vi "OnAxisPotential.vi"(1 "Requested Excitations":dbl[](array[numeric])=[0.0, 10.0, 10.0, 2.0, 20.0, 0.0, 0.0, 0.0, 0.0, 0.0, 0.0, 0.0, 0.0, 0.0, 0.0, 0.0, 0.0, 0.0, 0.0, 0.0, 0.0, 0.0], 2 "ComsolArray":dbl[][](array[numeric])=array1050x22[23100 elements], 3 "z (m)":dbl[](array[numeric])=[-0.5004, -0.4999, -0.4995, -0.499, -0.4985, -0.498, -0.4975, -0.4971, -0.4966, -0.4961, -0.4956, -0.4952, -0.4947, -0.4942, -0.4937, -0.4933, -0.4928, -0.4923, -0.4918, -0.4913, -0.4909, -0.4904, -0.4899, -0.4894, -0.489, -0.4885, -0.488, -0.4875, -0.4871, -0.4866, -0.4861, -0.4856, -0.4851, -0.4847, -0.4842, -0.4837, -0.4832, -0.4828, -0.4823, -0.4818, -0.4813, -0.4809, -0.4804, -0.4799, -0.4794, -0.4789, -0.4785, -0.478, -0.4775, -0.477, -0.4766, -0.4761, -0.4756, -0.4751, -0.4747, -0.4742, -0.4737, -0.4732, -0.4727, -0.4723, -0.4718, -0.4713, -0.4708, -0.4704, -0.4699, -0.4694, -0.4689, -0.4685, -0.468, -0.4675, -0.467, -0.4665, -0.4661, -0.4656, -0.4651, -0.4646, -0.4642, -0.4637, -0.4632, -0.4627, -0.4623, -0.4618, -0.4613, -0.4608, -0.4604, -0.4599, -0.4594, -0.4589, -0.4584, -0.458, -0.4575, -0.457, -0.4565, -0.4561, -0.4556, -0.4551, -0.4546, -0.4542, -0.4537, -0.4532, -0.4527, -0.4522, -0.4518, -0.4513, -0.4508, -0.4503, -0.4499, -0.4494, -0.4489, -0.4484, -0.448, -0.4475, -0.447, -0.4465, -0.446, -0.4456, -0.4451, -0.4446, -0.4441, -0.4437, -0.4432, -0.4427, -0.4422, -0.4418, -0.4413, -0.4408, -0.4403, -0.4398, -0.4394, -0.4389, -0.4384, -0.4379, -0.4375, -0.437, -0.4365, -0.436, -0.4356, -0.4351, -0.4346, -0.4341, -0.4336, -0.4332, -0.4327, -0.4322, -0.4317, -0.4313, -0.4308, -0.4303, -0.4298, -0.4294, -0.4289, -0.4284, -0.4279, -0.4274, -0.427, -0.4265, -0.426, -0.4255, -0.4251, -0.4246, -0.4241, -0.4236, -0.4232, -0.4227, -0.4222, -0.4217, -0.4212, -0.4208, -0.4203, -0.4198, -0.4193, -0.4189, -0.4184, -0.4179, -0.4174, -0.417, -0.4165, -0.416, -0.4155, -0.415, -0.4146, -0.4141, -0.4136, -0.4131, -0.4127, -0.4122, -0.4117, -0.4112, -0.4108, -0.4103, -0.4098, -0.4093, -0.4089, -0.4084, -0.4079, -0.4074, -0.4069, -0.4065, -0.406, -0.4055, -0.405, -0.4046, -0.4041, -0.4036, -0.4031, -0.4027, -0.4022, -0.4017, -0.4012, -0.4007, -0.4003, -0.3998, -0.3993, -0.3988, -0.3984, -0.3979, -0.3974, -0.3969, -0.3965, -0.396, -0.3955, -0.395, -0.3945, -0.3941, -0.3936, -0.3931, -0.3926, -0.3922, -0.3917, -0.3912, -0.3907, -0.3903, -0.3898, -0.3893, -0.3888, -0.3883, -0.3879, -0.3874, -0.3869, -0.3864, -0.386, -0.3855, -0.385, -0.3845, -0.3841, -0.3836, -0.3831, -0.3826, -0.3821, -0.3817, -0.3812, -0.3807, -0.3802, -0.3798, -0.3793, -0.3788, -0.3783, -0.3779, -0.3774, -0.3769, -0.3764, -0.3759, -0.3755, -0.375, -0.3745, -0.374, -0.3736, -0.3731, -0.3726, -0.3721, -0.3717, -0.3712, -0.3707, -0.3702, -0.3697, -0.3693, -0.3688, -0.3683, -0.3678, -0.3674, -0.3669, -0.3664, -0.3659, -0.3655, -0.365, -0.3645, -0.364, -0.3635, -0.3631, -0.3626, -0.3621, -0.3616, -0.3612, -0.3607, -0.3602, -0.3597, -0.3593, -0.3588, -0.3583, -0.3578, -0.3573, -0.3569, -0.3564, -0.3559, -0.3554, -0.355, -0.3545, -0.354, -0.3535, -0.3531, -0.3526, -0.3521, -0.3516, -0.3512, -0.3507, -0.3502, -0.3497, -0.3492, -0.3488, -0.3483, -0.3478, -0.3473, -0.3469, -0.3464, -0.3459, -0.3454, -0.345, -0.3445, -0.344, -0.3435, -0.343, -0.3426, -0.3421, -0.3416, -0.3411, -0.3407, -0.3402, -0.3397, -0.3392, -0.3388, -0.3383, -0.3378, -0.3373, -0.3368, -0.3364, -0.3359, -0.3354, -0.3349, -0.3345, -0.334, -0.3335, -0.333, -0.3326, -0.3321, -0.3316, -0.3311, -0.3306, -0.3302, -0.3297, -0.3292, -0.3287, -0.3283, -0.3278, -0.3273, -0.3268, -0.3264, -0.3259, -0.3254, -0.3249, -0.3244, -0.324, -0.3235, -0.323, -0.3225, -0.3221, -0.3216, -0.3211, -0.3206, -0.3202, -0.3197, -0.3192, -0.3187, -0.3182, -0.3178, -0.3173, -0.3168, -0.3163, -0.3159, -0.3154, -0.3149, -0.3144, -0.314, -0.3135, -0.313, -0.3125, -0.3121, -0.3116, -0.3111, -0.3106, -0.3101, -0.3097, -0.3092, -0.3087, -0.3082, -0.3078, -0.3073, -0.3068, -0.3063, -0.3059, -0.3054, -0.3049, -0.3044, -0.3039, -0.3035, -0.303, -0.3025, -0.302, -0.3016, -0.3011, -0.3006, -0.3001, -0.2997, -0.2992, -0.2987, -0.2982, -0.2977, -0.2973, -0.2968, -0.2963, -0.2958, -0.2954, -0.2949, -0.2944, -0.2939, -0.2935, -0.293, -0.2925, -0.292, -0.2915, -0.2911, -0.2906, -0.2901, -0.2896, -0.2892, -0.2887, -0.2882, -0.2877, -0.2873, -0.2868, -0.2863, -0.2858, -0.2853, -0.2849, -0.2844, -0.2839, -0.2834, -0.283, -0.2825, -0.282, -0.2815, -0.2811, -0.2806, -0.2801, -0.2796, -0.2791, -0.2787, -0.2782, -0.2777, -0.2772, -0.2768, -0.2763, -0.2758, -0.2753, -0.2749, -0.2744, -0.2739, -0.2734, -0.2729, -0.2725, -0.272, -0.2715, -0.271, -0.2706, -0.2701, -0.2696, -0.2691, -0.2687, -0.2682, -0.2677, -0.2672, -0.2667, -0.2663, -0.2658, -0.2653, -0.2648, -0.2644, -0.2639, -0.2634, -0.2629, -0.2625, -0.262, -0.2615, -0.261, -0.2605, -0.2601, -0.2596, -0.2591, -0.2586, -0.2582, -0.2577, -0.2572, -0.2567, -0.2563, -0.2558, -0.2553, -0.2548, -0.2544, -0.2539, -0.2534, -0.2529, -0.2524, -0.252, -0.2515, -0.251, -0.2505, -0.2501, -0.2496, -0.2491, -0.2486, -0.2482, -0.2477, -0.2472, -0.2467, -0.2462, -0.2458, -0.2453, -0.2448, -0.2443, -0.2439, -0.2434, -0.2429, -0.2424, -0.242, -0.2415, -0.241, -0.2405, -0.24, -0.2396, -0.2391, -0.2386, -0.2381, -0.2377, -0.2372, -0.2367, -0.2362, -0.2358, -0.2353, -0.2348, -0.2343, -0.2338, -0.2334, -0.2329, -0.2324, -0.2319, -0.2315, -0.231, -0.2305, -0.23, -0.2296, -0.2291, -0.2286, -0.2281, -0.2276, -0.2272, -0.2267, -0.2262, -0.2257, -0.2253, -0.2248, -0.2243, -0.2238, -0.2234, -0.2229, -0.2224, -0.2219, -0.2214, -0.221, -0.2205, -0.22, -0.2195, -0.2191, -0.2186, -0.2181, -0.2176, -0.2172, -0.2167, -0.2162, -0.2157, -0.2153, -0.2148, -0.2143, -0.2138, -0.2133, -0.2129, -0.2124, -0.2119, -0.2114, -0.211, -0.2105, -0.21, -0.2095, -0.2091, -0.2086, -0.2081, -0.2076, -0.2071, -0.2067, -0.2062, -0.2057, -0.2052, -0.2048, -0.2043, -0.2038, -0.2033, -0.2029, -0.2024, -0.2019, -0.2014, -0.2009, -0.2005, -0.2, -0.1995, -0.199, -0.1986, -0.1981, -0.1976, -0.1971, -0.1967, -0.1962, -0.1957, -0.1952, -0.1947, -0.1943, -0.1938, -0.1933, -0.1928, -0.1924, -0.1919, -0.1914, -0.1909, -0.1905, -0.19, -0.1895, -0.189, -0.1885, -0.1881, -0.1876, -0.1871, -0.1866, -0.1862, -0.1857, -0.1852, -0.1847, -0.1843, -0.1838, -0.1833, -0.1828, -0.1823, -0.1819, -0.1814, -0.1809, -0.1804, -0.18, -0.1795, -0.179, -0.1785, -0.1781, -0.1776, -0.1771, -0.1766, -0.1761, -0.1757, -0.1752, -0.1747, -0.1742, -0.1738, -0.1733, -0.1728, -0.1723, -0.1719, -0.1714, -0.1709, -0.1704, -0.1699, -0.1695, -0.169, -0.1685, -0.168, -0.1676, -0.1671, -0.1666, -0.1661, -0.1657, -0.1652, -0.1647, -0.1642, -0.1637, -0.1633, -0.1628, -0.1623, -0.1618, -0.1614, -0.1609, -0.1604, -0.1599, -0.1595, -0.159, -0.1585, -0.158, -0.1576, -0.1571, -0.1566, -0.1561, -0.1556, -0.1552, -0.1547, -0.1542, -0.1537, -0.1533, -0.1528, -0.1523, -0.1518, -0.1514, -0.1509, -0.1504, -0.1499, -0.1494, -0.149, -0.1485, -0.148, -0.1475, -0.1471, -0.1466, -0.1461, -0.1456, -0.1452, -0.1447, -0.1442, -0.1437, -0.1432, -0.1428, -0.1423, -0.1418, -0.1413, -0.1409, -0.1404, -0.1399, -0.1394, -0.139, -0.1385, -0.138, -0.1375, -0.137, -0.1366, -0.1361, -0.1356, -0.1351, -0.1347, -0.1342, -0.1337, -0.1332, -0.1328, -0.1323, -0.1318, -0.1313, -0.1308, -0.1304, -0.1299, -0.1294, -0.1289, -0.1285, -0.128, -0.1275, -0.127, -0.1266, -0.1261, -0.1256, -0.1251, -0.1246, -0.1242, -0.1237, -0.1232, -0.1227, -0.1223, -0.1218, -0.1213, -0.1208, -0.1204, -0.1199, -0.1194, -0.1189, -0.1185, -0.118, -0.1175, -0.117, -0.1165, -0.1161, -0.1156, -0.1151, -0.1146, -0.1142, -0.1137, -0.1132, -0.1127, -0.1123, -0.1118, -0.1113, -0.1108, -0.1103, -0.1099, -0.1094, -0.1089, -0.1084, -0.108, -0.1075, -0.107, -0.1065, -0.1061, -0.1056, -0.1051, -0.1046, -0.1041, -0.1037, -0.1032, -0.1027, -0.1022, -0.1018, -0.1013, -0.1008, -0.1003, -0.0999, -0.0994, -0.0989, -0.0984, -0.0979, -0.0975, -0.097, -0.0965, -0.096, -0.0956, -0.0951, -0.0946, -0.0941, -0.0937, -0.0932, -0.0927, -0.0922, -0.0917, -0.0913, -0.0908, -0.0903, -0.0898, -0.0894, -0.0889, -0.0884, -0.0879, -0.0875, -0.087, -0.0865, -0.086, -0.0855, -0.0851, -0.0846, -0.0841, -0.0836, -0.0832, -0.0827, -0.0822, -0.0817, -0.0813, -0.0808, -0.0803, -0.0798, -0.0793, -0.0789, -0.0784, -0.0779, -0.0774, -0.077, -0.0765, -0.076, -0.0755, -0.0751, -0.0746, -0.0741, -0.0736, -0.0731, -0.0727, -0.0722, -0.0717, -0.0712, -0.0708, -0.0703, -0.0698, -0.0693, -0.0689, -0.0684, -0.0679, -0.0674, -0.0669, -0.0665, -0.066, -0.0655, -0.065, -0.0646, -0.0641, -0.0636, -0.0631, -0.0627, -0.0622, -0.0617, -0.0612, -0.0608, -0.0603, -0.0598, -0.0593, -0.0588, -0.0584, -0.0579, -0.0574, -0.0569, -0.0565, -0.056, -0.0555, -0.055, -0.0546, -0.0541, -0.0536, -0.0531, -0.0526, -0.0522, -0.0517, -0.0512, -0.0507, -0.0503, -0.0498, -0.0493, -0.0488, -0.0484, -0.0479, -0.0474, -0.0469, -0.0464, -0.046, -0.0455, -0.045, -0.0445, -0.0441, -0.0436, -0.0431, -0.0426, -0.0422, -0.0417, -0.0412, -0.0407, -0.0402, -0.0398, -0.0393, -0.0388, -0.0383, -0.0379, -0.0374, -0.0369, -0.0364, -0.036, -0.0355, -0.035, -0.0345, -0.034, -0.0336, -0.0331, -0.0326, -0.0321, -0.0317, -0.0312, -0.0307, -0.0302, -0.0298, -0.0293, -0.0288, -0.0283, -0.0278, -0.0274, -0.0269, -0.0264, -0.0259, -0.0255, -0.025, -0.0245, -0.024, -0.0236, -0.0231, -0.0226, -0.0221, -0.0216, -0.0212, -0.0207, -0.0202, -0.0197, -0.0193, -0.0188, -0.0183, -0.0178, -0.0174, -0.0169, -0.0164, -0.0159, -0.0155, -0.015, -0.0145, -0.014, -0.0135, -0.0131, -0.0126, -0.0121, -0.0116, -0.0112, -0.0107, -0.0102, -0.0097, -0.0093, -0.0088, -0.0083, -0.0078, -0.0073, -0.0069, -0.0064, -0.0059, -0.0054, -0.005, -0.0045, -0.004, -0.0035, -0.0031, -0.0026, -0.0021, -0.0016, -0.0011, -0.0007, -0.0002], 4 "# electrodes":i32=22) -> (0 "XY Graph":cluster{"z (mm)":dbl[], dbl[]}(graph))   [LabVIEW 2018]
panel:
  in  "Excitations":dbl[](array[numeric])=[0.0, 10.0, 10.0, 2.0, 20.0, 0.0, 0.0, 0.0, 0.0, 0.0, 0.0, 0.0, 0.0, 0.0, 0.0, 0.0, 0.0, 0.0, 0.0, 0.0, 0.0, 0.0]
  # "This VI is called by PotentialEditor"
  # "If Requested does not contain correct number of electrodes,\nThen Excitations default to 0."
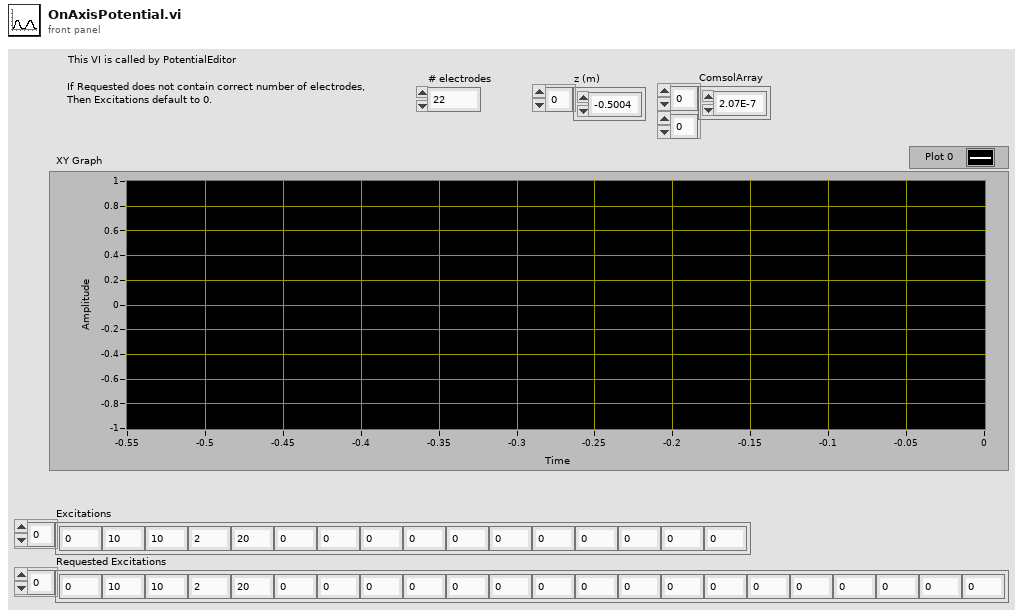
[diagram p1: front panel]
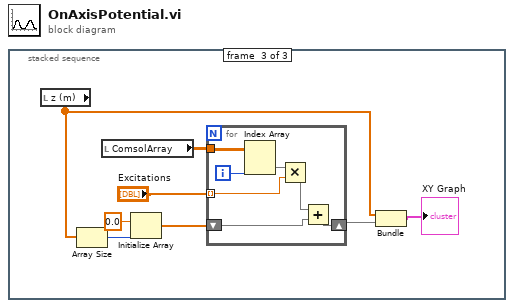
[diagram p0: block diagram]
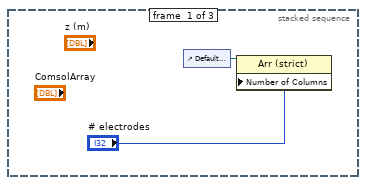
[diagram p2: hidden frame]
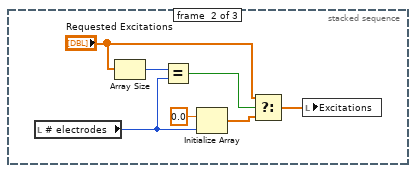
[diagram p3: hidden frame]
diagram:
  n1 = stacked-sequence {
    frame #0 {
      n2 = control-ref of="Default Excitations"() -> (w2:refnum<vi>)
      n3 = property class="Arr (strict)"(reference=w2, "Number of Columns"="# electrodes") -> ()  [unwired: 1 in, 2 out]
    }
    frame #1 {
      n4 = local read "# electrodes"() -> (w8:i32)
      n5 = Array Size(array="Requested Excitations") -> (size(s)=w7:i32)
      n6 = Equal?(x=w7, y=w8) -> (x = y?=w5:bool)
      n7 = Initialize Array(0.0 ("element"), w8) -> (w6:dbl[])
      n8 = Select(t="Requested Excitations", s=w5, f=w6) -> (s? t:f=w3:dbl[])
      n9 = local write "Excitations"(w3) -> ()
    }
    frame #2 {
      n10 = local read "z (m)"() -> (w11:dbl[])
      n11 = Array Size(array=w11) -> (size(s)=w15:i32)
      n12 = local read "ComsolArray"() -> (w17:dbl[][])
      n13 = Initialize Array(0.0 ("element"), w15) -> (w13:dbl[])
      n14 = for {
        tunnel: w17 -> [w24]
        tunnel: "Excitations" -> [w21] mode=indexing
        shift-right: [w18] -> w12
        shift-left: w13 -> [w20]
        i -> [w23]
        n15 = Index Array(array=w24, index (col)=w23) -> (element=w22:dbl[])  [unwired: 1 in]
        n16 = Multiply(x=w22, y=w21) -> (x*y=w19:dbl[])
        n17 = Add(x=w19, y=w20) -> (x+y=w18:dbl[])
      }
      n18 = Bundle("z (m)"=w11, w12) -> (→"XY Graph":cluster{"z (m)":dbl[], dbl[]})  [unwired: 1 in]
    }
  }
